vi "Close Phidget servos.vi"(1 "error in":errorcluster, 2 "Device In":i32) -> (0 "error out":errorcluster)   [LabVIEW 2014]
doc: "This VI will close the servos used in the ACT lab."
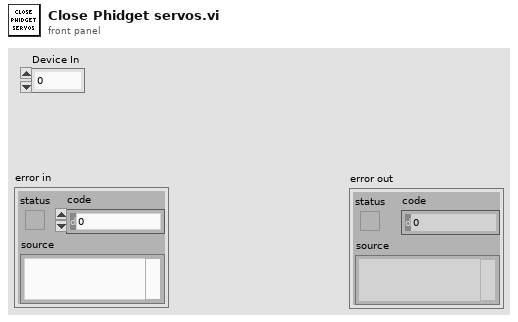
[diagram p1: front panel]
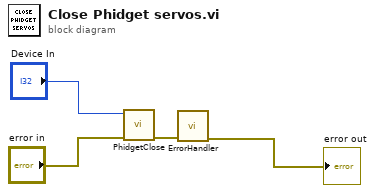
[diagram p0: block diagram]
diagram:
  n1 = call "PhidgetClose.vi"("error in"="error in", "Device In"="Device In") -> ("error out"=w3:errorcluster)  [unwired: 9 in]
  n2 = call "ErrorHandler.vi"("error in"=w3) -> ("error out"=→"error out":errorcluster)  [unwired: 9 in, 1 out]
